vi "dfd_Utility I64 x I32 .vi"(10 "y[I32]":i32, 11 "x[I64]":i64[](array[numeric])) -> (2 "x*y [Lo U32]":u32[](array[numeric]), 3 "x*y[Hi I64]":i64[](array[numeric]))   [LabVIEW 2017, in "NI_DigFilterLicensed.lvlib"]
uses:
  <vilib>/addons/Digital Filter Design/NI_DigFilterLicensed.lvlib
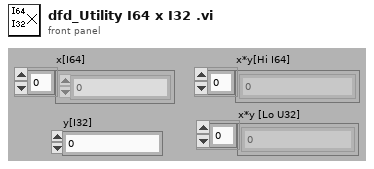
[diagram p1: front panel]
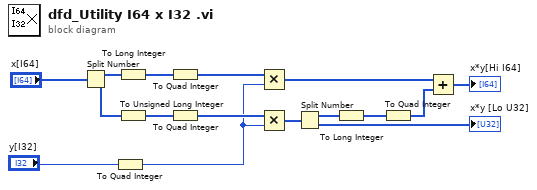
[diagram p0: block diagram]
diagram:
  n1 = Split Number(x="x[I64]") -> (hi(x)=w16:u32[], lo(x)=w15:u32[])
  n2 = To Quad Integer(1:"y[I32]") -> (0:w10:i64)
  n3 = To Long Integer(number=w16) -> (32bit integer=w14:i32[])
  n4 = To Unsigned Long Integer(number=w15) -> (unsigned 32bit integer=w13:u32[])
  n5 = To Quad Integer(1:w14) -> (0:w12:i64[])
  n6 = To Quad Integer(1:w13) -> (0:w11:i64[])
  n7 = Multiply(x=w12, y=w10) -> (x*y=w9:i64[])
  n8 = Multiply(x=w11, y=w10) -> (x*y=w6:i64[])
  n9 = Split Number(x=w6) -> (hi(x)=w5:u32[], lo(x)=→"x*y [Lo U32]":u32[])
  n10 = To Long Integer(number=w5) -> (32bit integer=w3:i32[])
  n11 = To Quad Integer(1:w3) -> (0:w4:i64[])
  n12 = Add(x=w9, y=w4) -> (x+y=→"x*y[Hi I64]":i64[])
